vi "Write Frame.vi"(7 "OpCode":T1, 8 "error in (no error)":errorcluster, 9 "Timeout ms":i32, 10 "Payload":string, 11 "WebSocket Client in":refnum<class "WebSocket Client.lvclass">) -> (0 "error out":errorcluster, 1 "Remaining  Timeout":i32, 3 "WebSocket Client out":refnum<class "WebSocket Client.lvclass">)   [LabVIEW 2020, in "HTTP Server.lvlib" / "WebSocket Client.lvclass"]
uses:
  WebSocket Client.lvclass
  WebSocket Client.lvclass/WebSocket Client.ctl
  OpCode.ctl
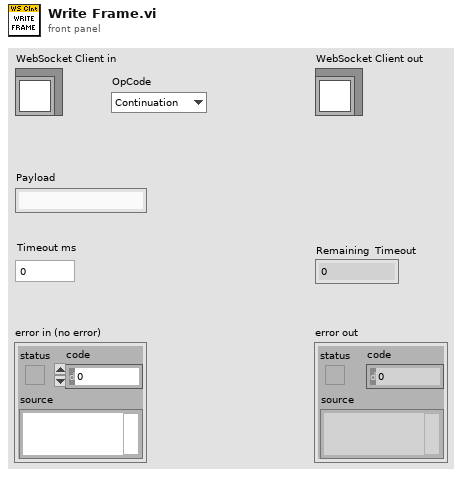
[diagram p1: front panel]
types:
  T1 = typedef "HTTP Server.lvlib/WebSocket Client.lvclass/OpCode.ctl" = enum8{"Continuation", "Text", "Binary", "Reserved3", "Reserved4", "Reserved5", "Reserved6", "Reserved7", "Close", "Ping", "Pong", "ReservedB", "ReservedC", "ReservedD", "ReservedE", "ReservedF"}
  T2 = typedef "HTTP Server.lvlib/WebSocket Client.lvclass/Message Frame.ctl" = cluster{"FIN":bool, "RSV1":bool, "RSV2":bool, "RSV3":bool, "MASK":bool, "OpCode":T1, "Length":u64, "MaskingKey":u8[], "Payload":string}
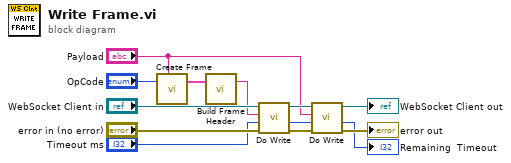
[diagram p0: block diagram]
diagram:
  n1 = call "Create Frame.vi"("OpCode"="OpCode", "Payload"="Payload") -> ("Message Frame"=w11:T2)  [unwired: 5 in]
  n2 = call "Build Frame Header.vi"("Message Frame"=w11) -> ("Header"=w7:string)  [unwired: 6 in]
  n3 = call "Do Write.vi"("error in (no error)"="error in (no error)", "Timeout ms"="Timeout ms", "Data"=w7, "WebSocket Client in"="WebSocket Client in") -> ("error out"=w10:errorcluster, "Remaining  Timeout"=w2:i32, "WebSocket Client out"=w5:refnum<class "WebSocket Client.lvclass">)  [unwired: 5 in]
  n4 = call "Do Write.vi"("error in (no error)"=w10, "Timeout ms"=w2, "Data"="Payload", "WebSocket Client in"=w5) -> ("error out"=→"error out":errorcluster, "Remaining  Timeout"=→"Remaining  Timeout":i32, "WebSocket Client out"=→"WebSocket Client out":refnum<class "WebSocket Client.lvclass">)  [unwired: 5 in]
